vi "Get Data For Intensity Graph.vi"(8 "error in":errorcluster, 9 "Secondary channel":dbl, 10 "Primary channel":dbl, 11 "Scan Driver in":refnum<class "Scan Driver.lvclass">) -> (0 "error out":errorcluster, 1 "Secondary graph points":T2, 2 "Primary graph points":T2, 3 "Scan Driver out":refnum<class "Scan Driver.lvclass">)   [LabVIEW 2017, in "Scan Driver.lvclass"]
doc: "Build and return the updated scan graph from the data store."
uses:
  Scan Driver.lvclass
  Instruments/Utility Classes/Readable/X.ctl
  Scan Driver.lvclass/Scan Driver.ctl
  Scanners/Scanner/Scanner.lvclass
  File IO/File IO.lvclass
  Instruments/Utility Classes/Readable/Readable.lvclass
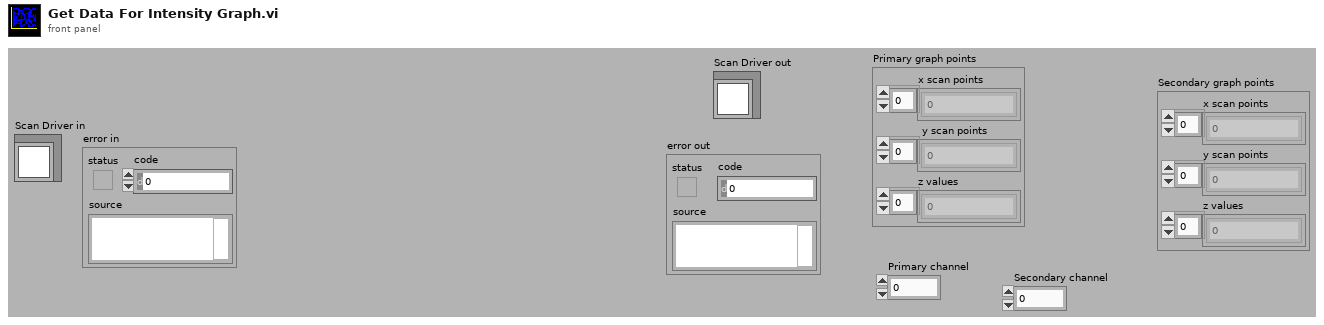
[diagram p1: front panel]
types:
  T1 = typedef "Readable.lvclass/X.ctl" = dbl
  T2 = cluster{"x scan points":T1[], "y scan points":T1[], "z values":T1[]}
  T3 = typedef "Readable.lvclass/Data Store.ctl" = T4[][]
  T4 = typedef "Readable.lvclass/Data Point.ctl" = cluster{"t":T5, "x":T1}
  T5 = typedef "Readable.lvclass/Time.ctl" = timestamp
  T6 = cluster{"Data Points":T1[], "Data Points":T1[], "Data Points":T1[]}
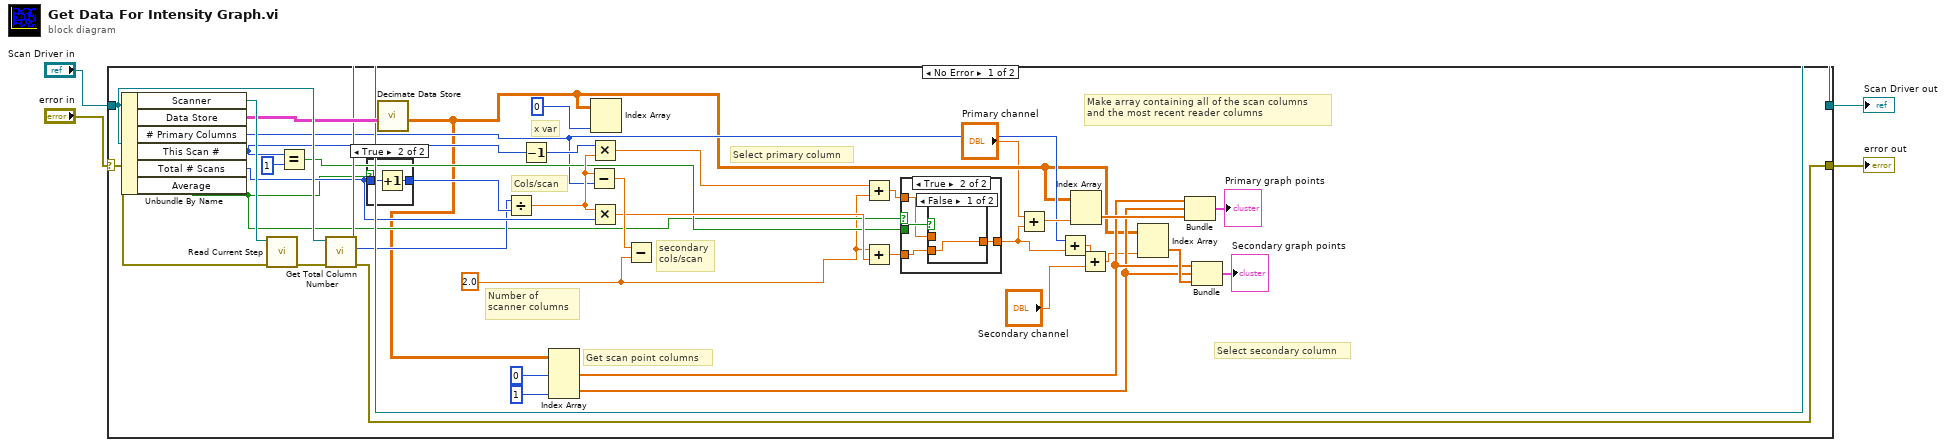
[diagram p0: block diagram]
diagram:
  n1 = case shown="No Error" "error in" {
    selector: "error in" -> [w42 w55]
    tunnel: "Scan Driver in" -> [w41 w54]
    tunnel: [w36 w55] -> w3
    tunnel: [w38 w54] -> w1
    frame No Error {
      w13 = 2.0 ("t")
      # "Make array containing all of the scan columns\nand the most recent reader columns"
      # "secondary\ncols/scan"
      # "Get scan point columns"
      # "Number of \nscanner columns"
      # "Select secondary column"
      # "Select primary column"
      # "Cols/scan"
      # "x var"
      n2 = Unbundle By Name(w41) -> ("Scanner"=w43:refnum<class "Scanner.lvclass">, "Data Store"=w39:T3, "# Primary Columns"=w11:u32, "This Scan #"=w33:u32, "Total # Scans"=w35:u32, "Average"=w17:bool)
      n3 = call-dynamic "Read Current Step.vi"("error in (no error)"=w42, "Scanner.lvclass in"=w43) -> ("error out"=w40:errorcluster)  [unwired: 5 in, 4 out]
      n4 = Equal?(x=w33, y=1) -> (x = y?=w18:bool)
      n5 = call "Get Total Column Number.vi"("error in (no error)"=w40, "Scan Driver.lvclass"=w41) -> ("error out"=w36:errorcluster, "# of Columns"=w32:i32, "Scan Driver.lvclass"=w38:refnum<class "Scan Driver.lvclass">)  [unwired: 7 in]
      n6 = case shown="True" w17 {
        tunnel: [w51 w53] -> w37
        tunnel: w35 -> [w51 w52]
        frame False {
        }
        frame True {
          n7 = Increment(x=w52) -> (x+1=w53:u32)
        }
      }
      n8 = call "Decimate Data Store.vi"("Data Store"=w39) -> ("Data Points"=w10:T1[][])  [unwired: 9 in, 1 out]
      n9 = Divide(x=w32, y=w37) -> (x/y=w29:dbl)
      n10 = Decrement(x=w33) -> (x-1=w30:u32)
      n11 = Index Array(array=w10, index (col) #1=0 ("index"), index (col) #2=1 ("index (col)")) -> (element #1=w15:T1[], element #2=w14:T1[])  [unwired: 2 in]
      n12 = Subtract(x=w29, y=w11) -> (x-y=w28:dbl)
      n13 = Multiply(x=w30, y=w29) -> (x*y=w16:dbl)
      n14 = Multiply(x=w29, y=w35) -> (x*y=w19:dbl)
      n15 = Index Array(array=w10, index (col)=0) -> ()  [unwired: 1 in, 1 out]
      n16 = Subtract(x=w28, y=w13) -> ()  [unwired: 1 out]
      n17 = Add(x=w16, y=w13) -> (x+y=w26:dbl)
      n18 = Add(x=w13, y=w19) -> (x+y=w27:dbl)
      n19 = case shown="True" w17 {
        tunnel: w27 -> [_ w47]
        tunnel: w26 -> [w44 w46]
        tunnel: w18 -> [_ w48]
        tunnel: [w44 w45] -> w5
        frame False {
        }
        frame True {
          n20 = case shown="False" w48 {
            tunnel: w47 -> [w49 _]
            tunnel: w46 -> [_ w50]
            tunnel: [w49 w50] -> w45
            frame False {
            }
            frame True {
            }
          }
        }
      }
      n21 = Add(x="Primary channel", y=w5) -> (x+y=w12:dbl)
      n22 = Add(x=w11, y=w5) -> (x+y=w8:dbl)
      n23 = Index Array(array=w10, index (col)=w12) -> (element=w23:T1[])  [unwired: 1 in]
      n24 = Add(x=w8, y="Secondary channel") -> (x+y=w7:dbl)
      n25 = Index Array(array=w10, index (col)=w7) -> (element=w21:T1[])  [unwired: 1 in]
      n26 = Bundle("Data Points"=w15, "Data Points"=w14, "Data Points"=w23) -> (→"Primary graph points":T6)  [unwired: 1 in]
      n27 = Bundle("Data Points"=w15, "Data Points"=w14, "Data Points"=w21) -> (→"Secondary graph points":T6)  [unwired: 1 in]
    }
    frame Error {
    }
  }
  "error out" <- w3
  "Scan Driver out" <- w1
